vi "Scalar Element Benchmark.vi"() -> ()   [LabVIEW 2022 SP3]
uses:
  Enclave/Element.ctl
  Enclave/Lossless/Lossless.lvclass/Lossless.ctl
  Enclave/Enclave/Enclave.lvclass/Enclave.ctl
  Enclave/Lossless/Read.vi
  Enclave/Instantiate.vi
  Enclave/Read Lossless Class.vi
  Enclave/))Channel.vi
  Enclave/Enclave/Check Ready.vi
  Enclave/Enclave/Close.vi
  Enclave/Enclave/Enclave.lvclass
  Enclave/Enclave.lvlib
panel:
  out "Element":T1
  out "El / S":i32(graph)
  in  "stop":bool
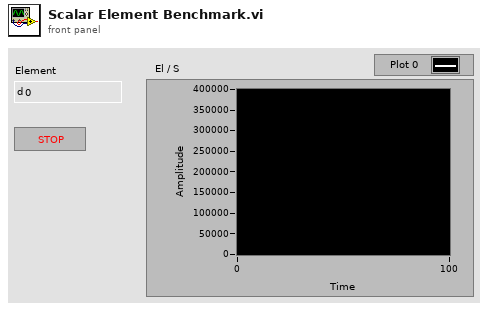
[diagram p1: front panel]
types:
  T1 = typedef "Enclave.lvlib/Element.ctl" = dbl
  T2 = typedef "Enclave.lvlib/))Channel.ctl" = refnum<queue>
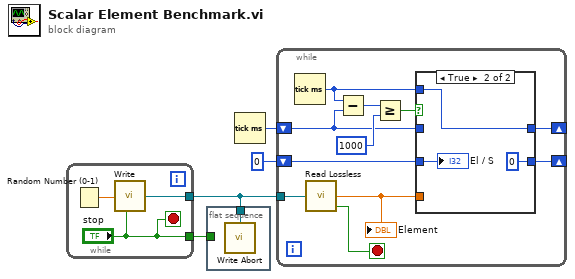
[diagram p0: block diagram]
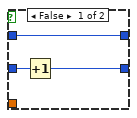
[diagram p2: hidden frame]
diagram:
  n1 = while {
    tunnel: [w6] -> w1
    tunnel: ["stop"] -> w2
    stop <- "stop" stop-if-true
    n2 = Random Number (0-1)() -> (number: 0 to 1=w7:dbl)
    n3 = call "Write.vi"("Element"=w7, "Close (F)"="stop") -> ("EnclaveChannel"=w6:T2)  [unwired: 5 in, 2 out]
  }
  n4 = flat-sequence {
    tunnel: w2 -> [_]
    tunnel: w1 -> [w8]
    frame #0 {
      n5 = call "Write Abort.vi"("EnclaveChannel"=w8) -> ()
    }
  }
  n6 = Tick Count (ms)() -> (millisecond timer value=w4:u32)
  n7 = while {
    tunnel: w1 -> [w19]
    shift-right: [w12] -> _
    shift-left: w4 -> [w15]
    shift-right: [w10] -> _
    shift-left: 0 -> [w11]
    stop <- w18 stop-if-true
    n8 = Tick Count (ms)() -> (millisecond timer value=w13:u32)
    n9 = call "Read Lossless.vi"("EnclaveChannel"=w19) -> ("Element"=w9:T1, "Closed?"=w18:bool)  [unwired: 6 in, 1 out]
    "Element" <- w9
    n10 = Subtract(x=w13, y=w15) -> (x-y=w17:u32)
    n11 = Greater Or Equal?(x=w17, y=u32 1000) -> (x >= y?=w14:bool)
    n12 = case shown="True" w14 {
      tunnel: w15 -> [w22 _]
      tunnel: w13 -> [_ w25]
      tunnel: [w22 w25] -> w12
      tunnel: w11 -> [w21 w24]
      tunnel: [w20 0] -> w10
      tunnel: w9 -> [_ _]
      frame False {
        n13 = Increment(x=w21) -> (x+1=w20:i32)
      }
      frame True {
        "El / S" <- w24
      }
    }
  }
